vi "Build.vi"(8 "error in (no error)":errorcluster, 11 "Build in":refnum<class "AB_DLL.lvclass">) -> (0 "error out":errorcluster, 1 "GeneratedFiles":path[](array[path]), 2 "GeneratedDirectories":path[](array[path]), 3 "Build out":refnum<class "AB_DLL.lvclass">, 4 "GeneratedFileGUIDs":string[](array[string]), 5 "OutputDirectory":path, 7 "Dependencies":T1[](array[typedef]))   [LabVIEW 2020, in "AB_DLL.lvclass"]
uses:
  <vilib>/AppBuilder/AB_Classes/DLL/AB_DLL.lvclass
  e:/builds/penguin/labview/branches/2020/dev/dist/vi.lib/AppBuilder/AB_Classes/Build/AB_Build.lvclass
  e:/builds/penguin/labview/branches/2020/dev/dist/vi.lib/AppBuilder/AB_Classes/TargetFile/AB_Targetfile.lvclass
  e:/builds/penguin/labview/branches/2020/dev/dist/vi.lib/AppBuilder/AB_Classes/Application/AB_Application.lvclass
  <vilib>/AppBuilder/AB_Dependency.ctl
  <vilib>/Utility/lvfile.llb/LVFileType.ctl
  <vilib>/AppBuilder/AB_Classes/DLL/AB_DLL.lvclass/AB_DLL.ctl
  <vilib>/AppBuilder/Engine/AB_Engine_RTDEP_LibDeploymentInfo.ctl
  <vilib>/AppBuilder/Engine/AB_Engine_RTDEP_Dep_Lib_Info.ctl
  <vilib>/AppBuilder/RW_Project/AB_RW_Project_EXE_ActiveX_Data.ctl
  <resource>/Framework/Providers/Common/provcom_StringGlobals.vi
  <vilib>/AppBuilder/AB_Classes/Application/AB_Application.lvclass
  <vilib>/AppBuilder/AB_Classes/Destination/AB_Destination.lvclass
  <vilib>/AppBuilder/AB_Classes/Build/AB_Build.lvclass
  <vilib>/AppBuilder/AB_Classes/TargetFile/AB_Targetfile.lvclass
  <vilib>/Utility/lvfile.llb/NI_FileType.lvlib
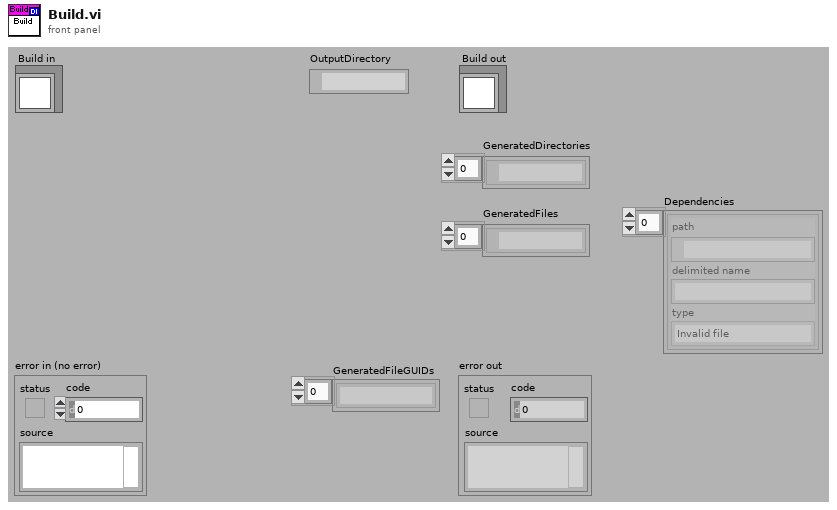
[diagram p1: front panel]
types:
  T1 = typedef "AB_Dependency.ctl" = cluster{"path":path, "delimited name":string, "type":T2}
  T2 = typedef "NI_FileType.lvlib/LVFileType.ctl" = enum32{"Invalid file", "Unknown type", "Instrument", "Control", "Polymorphic VI", "Project", "Library", "LVClass", "XControl", "XNode", "Shared library", ".NET assembly", "ActiveX interface", "CIN", "Run-time menu", "Palette menu", "Help file", "LLB", "XNode Edit Dependency", "Class Private Data Control", "Statechart", "MathScript .m file", "Ladder Diagram", "LVLibp", "XNode Build Dependency"}
  T3 = typedef "AB_Engine_RTDEP_LibDeploymentInfo.ctl" = cluster{"auto undeploy?":bool, "Array":T4[], "hide deployment dialog":bool}
  T4 = typedef "AB_Engine_RTDEP_Dep_Lib_Info.ctl" = cluster{"Library Path":path, "Target Name":string}
  T5 = typedef "AB_RW_Project_EXE_ActiveX_Data.ctl" = cluster{"Major Version":u16, "Minor Version":u16, "ProgID Prefix":string, "Obj CLSIDs":string[], "Enum CLSIDs":string[]}
  T6 = typedef "AB_Build.ctl" = cluster{"buildSpecName":string, "buildSpecDescription":string, "destinations":refnum<class "AB_Destination.lvclass">[], "exclusionOption":T7, "defaultLanguage":string, "supportedLanguages":string[], "excludedDirectories":path[], "buildContext":refnum<vi>, "buildObject":T8, "preview":bool, "programatic":bool, "progressBarEvents":T9, "userLog_Path":path, "preActionID":string, "preAction_Path":path, "postActionID":string, "postAction_Path":path, "eng_checkForBrokenVIs?":bool, "eng_verboseLinkerErrors?":bool, "localDest_Path":path, "targetDest_Path":path, "removeVIObject":u16, "cache":refnum<class "PreviewCache.lvclass">, "use cache":bool, "previewCache_ID":string, "buildCache_ID":string, "eng_TempLocalDest_Path":path, "eng_collectDependencies?":bool, "versionInfo":cluster{"buildVersion":cluster{"major":u16, "minor":u16, "patch":u16, "build":u16}, "autoIncrement":bool}, "eng_enableVIChecksums":bool}
  T7 = typedef "AB_Exclusion_Option.ctl" = cluster{"typedefs":bool, "polymorphicVIs":bool, "unusedLibraryItems":bool, "modifyLibraryFile":bool, "edit-timeDependencies":bool, "inlineVIs":bool, "dependent PPLs":bool, "dependent DLLs":bool}
  T8 = typedef "ItemRef.ctl" = u64
  T9 = typedef "provcom_ProgressBar_Events.ctl" = cluster{"newJob":refnum<user-event>, "newItem":refnum<user-event>, "errorMsg":T10, "cancel":refnum<user-event>}
  T10 = typedef "mxLvBuildError.ctl" = refnum<user-event>
  T11 = typedef "AB_DLL.ctl" = cluster{"delayOSMsg":bool, "includeHeaders":bool, "embeddedRTE":bool, "headerGUID":string, "libGUID":string, "compatibilityWith2011":bool, "includeTypeLibrary":bool, "privateExecutionSystem":bool}
  T12 = typedef "AB_Targetfile.ctl" = cluster{"targetfileName":string, "targetfileGUID":string, "enableDebugging":bool, "versionInfo":cluster{"productName":string, "legalCopyright":string, "companyName":string, "internalName":string, "fileDescription":string}, "eng_consolidatedTypeInfo":string, "fastFileFormat":bool, "eng_LEIFBuildData":u32, "versionIndependent":bool}
  T13 = typedef "AB_Application.ctl" = cluster{"INI_path":path, "INI_itemID":string, "INI_GUID":string, "aliasPath":path, "aliasItemID":string, "aliasGUID":string, "waitDebugging":bool, "copyErrors":bool, "useFFRTE":bool, "includeHWConfig":bool, "showHWConfig":bool, "winsec.certificate":string, "winsec.timestamp":string, "winsec.description":string, "winsec.manifestItemID":string, "winsec.manifestPath":path, "web service itemIDs":string[], "Embedded Server Configuration":T14, "Server Type":enum32{"NI Web Server", "Application Web Server"}}
  T14 = typedef "AB_Embedded_Server_Configuration.ctl" = cluster{"HTTP enabled?":bool, "HTTP port":i32, "HTTPS enabled?":bool, "HTTPS port":i32, "SSL certificate file":path}
  T15 = typedef "AB_Destination.ctl" = cluster{"destName":string, "path":path, "libraryName":string, "preserveHierarchy":bool, "eng_inBuild":bool, "eng_libraryReference":refnum<vi>, "eng_restictAddToNewLibrary":bool}
  T16 = enum32{"invalid OS target", "Mac OS", "Windows 3.1", "Windows 95/NT", "Solaris 1", "Solaris 2", "HP-UX", "PowerMAX", "Linux", "Irix", "Rhapsody", "BeOS", "AIX", "OSF1", "VxWorks", "PharLap", "Carbon", "RTX", "Windows x64", "Linux x64", "Mac OS X x64"}
  T17 = typedef "ABAPI Dist VI Proto Info New.ctl" = cluster{"cptm":string, "params":cluster{"name":string, "dir":enum32{"in", "out", "in/out", "length", "error-out"}, "inputIdx":i32, "outputIdx":i32, "passBy":i32, "lenInput":i32, "lenOutput":i32}[], "callingConv":i32, "name":string, "Description":string, "isCustomDesc":i32}
  T18 = enum32{"invalid CPU target", "Motorola 68K", "PowerPC", "Intel x86", "SPARC", "PA-RISC", "MIPS", "Alpha", "ARM", "AMD/Intel x64"}
  T19 = typedef "AB_Version_Info.ctl" = cluster{"PrivateBuild":string, "SpecialBuild":string, "LegalCopyright":string, "LegalTrademarks":string, "Comments":string, "FileDescription":string, "InternalName":string, "file version":cluster{"major":u16, "minor":u16, "patch":u16, "build":u16}, "ProductName":string, "FileType":u16, "CompanyName":string, "OriginalFilename":string}
  T20 = cluster{"appended path":path, "appended path":path, string, "App Memory Size":u32, "LVRT Target Dialog":i32, "pathAppShell":path, "AppFlags":u32, "activeX info out":T5, "Gen New AX Guids":bool, "defaultLanguage":string, "supportedLanguages":string[], "Lib Deployment Info":T3, "eng_consolidatedTypeInfo":string, "eng_LEIFBuildData":u32}
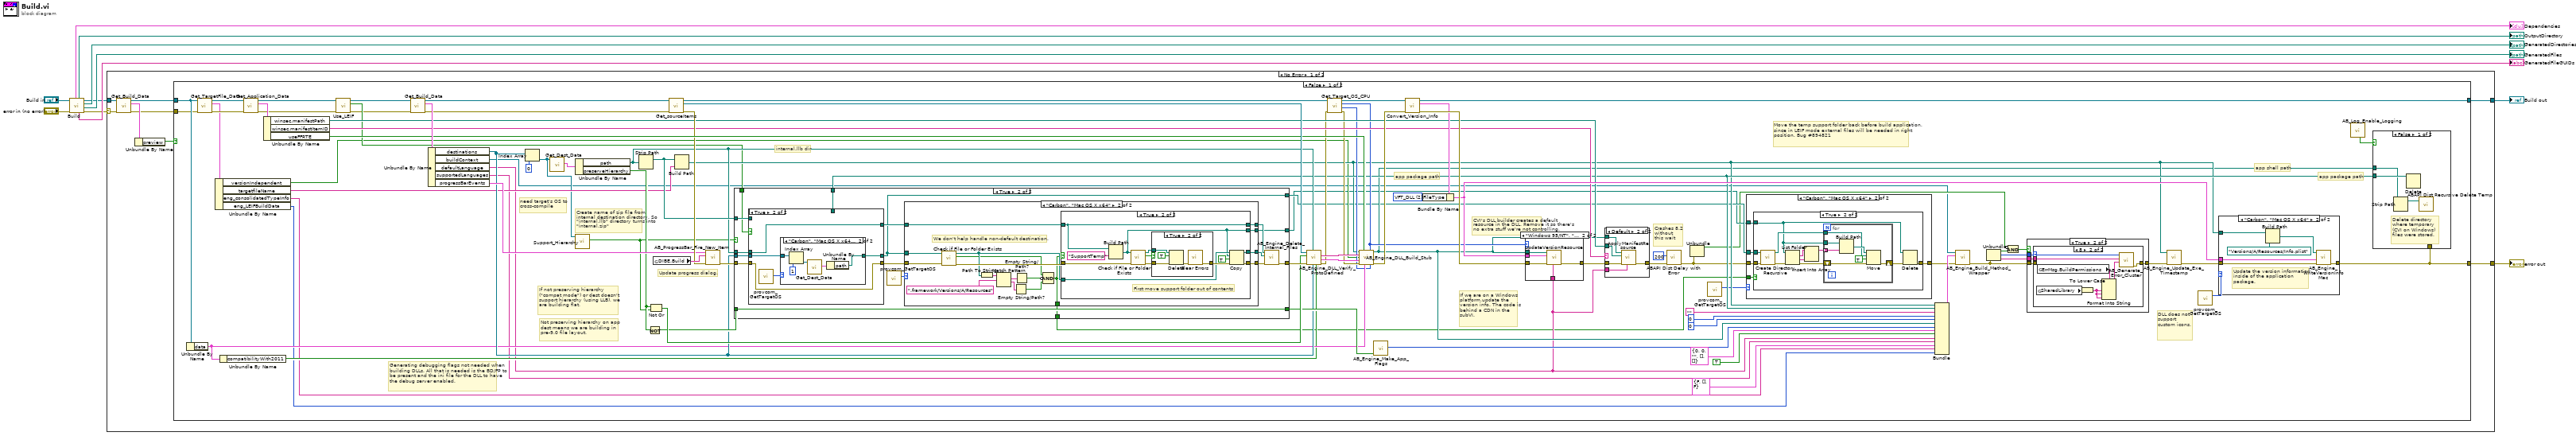
[diagram p0: block diagram]
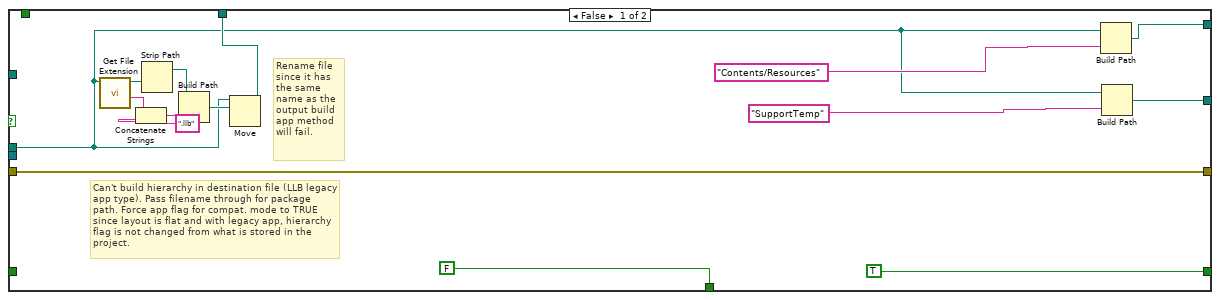
[diagram p6: hidden frame]
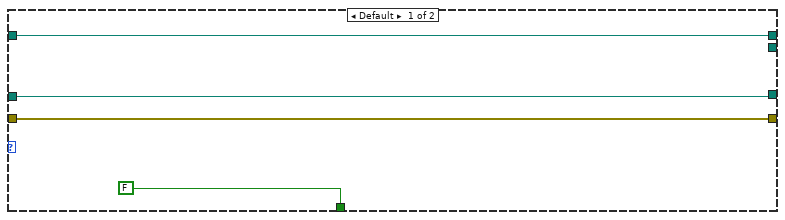
[diagram p7: hidden frame]
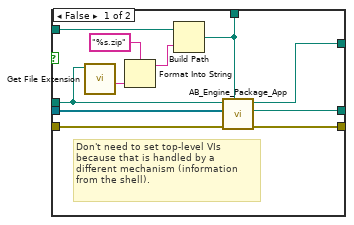
[diagram p10: hidden frame]
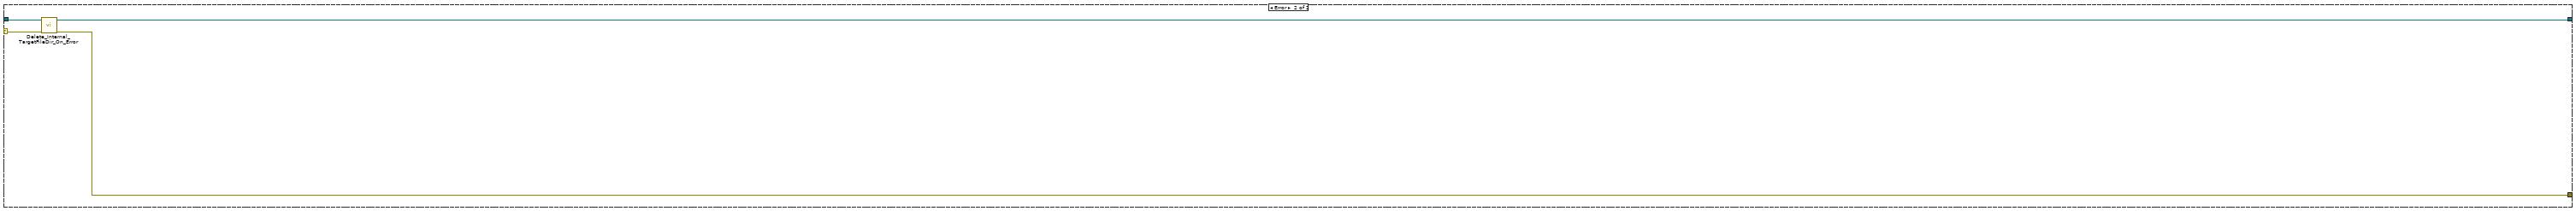
[diagram p17: hidden frame]
diagram:
  n1 = call-parent "Build.vi"("error in (no error)"="error in (no error)", "Build in"="Build in") -> ("error out"=w5:errorcluster, "GeneratedFiles"=→"GeneratedFiles":path[], "GeneratedDirectories"=→"GeneratedDirectories":path[], "Build out"=w4:refnum<class "AB_DLL.lvclass">, "GeneratedFileGUIDs"=→"GeneratedFileGUIDs":string[], "OutputDirectory"=→"OutputDirectory":path, "Dependencies"=→"Dependencies":T1[])  [unwired: 3 out]
  n2 = case shown="No Error" w5 {
    selector: w5 -> [w17 w266]
    tunnel: w4 -> [w18 w268]
    tunnel: [w12 w265] -> w3
    tunnel: [w13 w267] -> w2
    frame No Error {
      n3 = call <vilib>:"Get_Build_Data.vi"("error in (no error)"=w17, "Class in"=w18) -> ("error out"=w15:errorcluster, "data"=w19:T6, "Class out"=w14:refnum<class "AB_DLL.lvclass">)  [unwired: 7 out]
      n4 = Unbundle By Name(w19) -> ("preview"=w16:bool)
      n5 = case shown="False" w16 {
        tunnel: w15 -> [w67 w263]
        tunnel: w14 -> [w69 w264]
        tunnel: [w61 w264] -> w13
        tunnel: [w60 w263] -> w12
        frame False {
          w91 = u16 2 items=["VFT_UNKNOWN", "VFT_APP", "VFT_DLL", "VFT_DRV", "VFT_FONT", "VFT_VXD", "-", "VFT_STATIC_LIB"] ("FileType")
          # "Move the temp support folder back before build application, since in LEIF mode external files will be needed in right position. Bug #894821"
          # "need target's OS to cross-compile"
          # "app shell path"
          # "If not preserving hierarchy (\"compat mode\") or dest doesn't support hierarchy (using LLB), we are building flat."
          # "Not preserving hierarchy on app dest means we are building in pre-9.0 file layout."
          # "Create name of zip file from internal destination directory. So \"internal.llb\" directory turns into \"internal.zip\""
          # "internal.llb dir"
          # "app package path"
          # "app package path"
          # "Update progress dialog."
          # "CVI's DLL builder creates a default resource in the DLL. Remove it so there's no extra stuff we're not controlling."
          # "If we are on a Windows platform,update the version info. The code is behind a CDN in the subVI."
          # "Generating debugging flags not needed when building DLLs. All that is needed is the BD/FP to be present and the ini file for the DLL to have the debug server enabled."
          # "Crashes 8.2 without\nthis wait"
          # "DLL does not support custom icons."
          n6 = Unbundle By Name(w69) -> ("data"=w63:T11)
          n7 = call <vilib>:"Get_TargetFile_Data.vi"("error in (no error)"=w67, "AB_Targetfile in"=w69) -> ("error out"=w66:errorcluster, "data"=w65:T12, "AB_Targetfile out"=w68:refnum<class "AB_DLL.lvclass">)  [unwired: 7 in]
          n8 = Unbundle By Name(w65) -> ("versionIndependent"=w31:bool, "targetfileName"=w64:string, "eng_consolidatedTypeInfo"=w42:string, "eng_LEIFBuildData"=w32:u32)
          n9 = Unbundle By Name(w63) -> ("compatibilityWith2011"=w62:bool)
          n10 = call <vilib>:"Get_Application_Data.vi"("error in (no error)"=w66, "AB_Application in"=w68) -> ("error out"=w34:errorcluster, "data"=w107:T13, "AB_Application out"=w36:refnum<class "AB_DLL.lvclass">)  [unwired: 7 out]
          n11 = Unbundle By Name(w107) -> ("winsec.manifestPath"=w80:path, "winsec.manifestItemID"=w77:string, "useFFRTE"=w97:bool)
          n12 = call <vilib>:"Use_LEIF.vi"("error in (no error)"=w34, "AB_Targetfile in"=w36) -> ("error out"=w33:errorcluster, "use LEIF?"=w37:bool, "AB_Targetfile out"=w35:refnum<class "AB_DLL.lvclass">)  [unwired: 7 in]
          n13 = call <vilib>:"Get_Build_Data.vi"("error in (no error)"=w33, "Class in"=w35) -> ("error out"=w29:errorcluster, "data"=w106:T6, "Class out"=w30:refnum<class "AB_DLL.lvclass">)  [unwired: 7 out]
          n14 = Unbundle By Name(w106) -> ("destinations"=w70:refnum<class "AB_Destination.lvclass">[], "buildContext"=w20:refnum<vi>, "defaultLanguage"=w44:string, "supportedLanguages"=w43:string[], "progressBarEvents"=w88:T9)
          n15 = Index Array(array=w70, index=0) -> (element=w59:refnum<class "AB_Destination.lvclass">)
          n16 = call <vilib>:"Get_Dest_Data.vi"("Class in"=w59) -> ("destName"=w104:T15)  [unwired: 1 in, 9 out]
          n17 = call-dynamic "Support_Hierarchy.vi"("AB_Destination in"=w59) -> ("support hierarchy"=w73:bool)  [unwired: 1 in, 9 out]
          n18 = Unbundle By Name(w104) -> ("path"=w75:path, "preserveHierarchy"=w74:bool)
          n19 = Strip Path(path=w75) -> (stripped path=w81:path)  [unwired: 1 out]
          n20 = Not(x=w74) -> (.not. x?=w72:bool)
          n21 = Not Or(1:w73, 2:w74) -> (0:w76:bool)
          n22 = global read "provcom_StringGlobals.vi" "DIBE.Build"() -> (w90:string)
          n23 = call <vilib>:"Get_sourceItems.vi"("error in (no error)"=w29, "Class in"=w30) -> ("error out"=w89:errorcluster, "sourceItems"=w100:refnum<class "AB_Source.lvclass">[], "Class out"=w58:refnum<class "AB_DLL.lvclass">)  [unwired: 7 out]
          n24 = Build Path(base path=w81, name or relative path=w64) -> (appended path=w50:path)
          n25 = call <vilib>:"AB_ProgressBar_Fire_New_Item.vi"("error in (no error)"=w89, "Label"=w90, "progressBarEvents in"=w88) -> ("error out"=w83:errorcluster)  [unwired: 8 out]
          n26 = case shown="True" w73 {
            tunnel: w83 -> [w159 w176]
            tunnel: [w159 w170] -> w82
            tunnel: w75 -> [w145 w173]
            tunnel: w81 -> [_ w175]
            tunnel: [w151 w174] -> w51
            tunnel: w72 -> [_ w172]
            tunnel: [TRUE w172] -> w71
            tunnel: w70 -> [_ w171]
            tunnel: w37 -> [_ w169]
            tunnel: [w146 w164] -> w25
            tunnel: [w147 w161] -> w26
            tunnel: [FALSE ("file or folder exists?") w160] -> w24
            frame False {
              # "Rename file since it has the same name as the output build app method will fail."
              # "Can't build hierarchy in destination file (LLB legacy app type). Pass filename through for package path. Force app flag for compat. mode to TRUE since layout is flat and with legacy app, hierarchy flag is not changed from what is stored in the project."
              n27 = call <vilib>:"Get File Extension.vi"("file"=w145) -> ("filename without extension"=w157:string, "dup file"=w155:path)  [unwired: 1 in, 8 out]
              n28 = Concatenate Strings(w157, ".llb" ("string")) -> (w154:string)
              n29 = Strip Path(path=w155) -> (stripped path=w153:path)  [unwired: 1 out]
              n30 = Build Path(base path=w153, name or relative path=w154) -> (appended path=w152:path)
              n31 = Move(source path=w145, 10:w152) -> (3:w151:path)  [unwired: 1 in, 4 out]
              n32 = Build Path(base path=w145, name or relative path="Contents/Resources") -> (appended path=w147:path)
              n33 = Build Path(base path=w145, name or relative path="SupportTemp") -> (appended path=w146:path)
            }
            frame True {
              n34 = case shown="True" w169 {
                tunnel: w176 -> [w229 w234]
                tunnel: w175 -> [w225 _]
                tunnel: [w224 _] -> w174
                tunnel: [w221 w234] -> w162
                tunnel: w173 -> [w223 w230]
                tunnel: w171 -> [w222 w232]
                tunnel: [w220 w230] -> w167
                tunnel: [w219 w231] -> w161
                frame False {
                  # "Don't need to set top-level VIs because that is handled by a different mechanism (information from the shell)."
                  n35 = call <vilib>:"Get File Extension.vi"("file"=w223) -> ("filename without extension"=w228:string)  [unwired: 1 in, 9 out]
                  n36 = Format Into String(format string="%s.zip", w228) -> (resulting string=w227:string)  [unwired: 2 in, 1 out]
                  n37 = Build Path(base path=w225, name or relative path=w227) -> (appended path=w224:path)
                  n38 = call <vilib>:"AB_Engine_Package_App.vi"("application package path"=w224, "error in (no error)"=w229, "destinations"=w222, "internal directory"=w223) -> ("error out"=w221:errorcluster, "support dir"=w219:path, "dup internal directory"=w220:path)  [unwired: 1 in, 4 out]
                }
                frame True {
                  n39 = call <resource>:"provcom_GetTargetOS.vi"() -> ("App.TargetOS"=w233:T16)  [unwired: 11 out]
                  n40 = case shown="\"Carbon\", \"Mac OS X x64\"" w233 {
                    tunnel: w232 -> [_ w236]
                    tunnel: [_ w235] -> w231
                    frame Default {
                    }
                    frame "Carbon", "Mac OS X x64" {
                      n41 = Index Array(array=w236, index=1) -> (element=w239:refnum<class "AB_Destination.lvclass">)
                      n42 = call <vilib>:"Get_Dest_Data.vi"("Class in"=w239) -> ("destName"=w238:T15)  [unwired: 1 in, 9 out]
                      n43 = Unbundle By Name(w238) -> ("path"=w235:path)
                    }
                  }
                }
              }
              n44 = call <resource>:"provcom_GetTargetOS.vi"() -> ("App.TargetOS"=w163:T16)  [unwired: 11 out]
              n45 = case shown="\"Carbon\", \"Mac OS X x64\"" w163 {
                tunnel: [w178 w197] -> w168
                tunnel: w167 -> [w180 w196]
                tunnel: [w180 w195] -> w166
                tunnel: [w179 w194] -> w165
                tunnel: [_ w193] -> w164
                tunnel: w162 -> [w178 w192]
                tunnel: w161 -> [w179 w191]
                tunnel: [FALSE ("file or folder exists?") w184] -> w160
                frame Default {
                }
                frame "Carbon", "Mac OS X x64" {
                  # "We don't help handle non-default destination."
                  n46 = call <vilib>:"Check if File or Folder Exists.vi"("error in (no error)"=w192, "path"=w191) -> ("error out"=w190:errorcluster, "file or folder exists?"=w185:bool, "dup path"=w186:path)  [unwired: 7 in]
                  n47 = Path To String(path=w186) -> (string=w189:string)
                  n48 = Match Pattern(string=w189, regular expression=".framework/Versions/A/Resources") -> (match substring=w187:string, after substring=w183:string)  [unwired: 1 in, 2 out]
                  n49 = Empty String/Path?(string/path=w183) -> (empty?=w182:bool)
                  n50 = Empty String/Path?(string/path=w187) -> (empty?=w181:bool)
                  n51 = Compound Arithmetic op=AND(w185, invert w181, w182) -> (w184:bool)
                  n52 = case shown="True" w184 {
                    tunnel: w190 -> [w198 w201]
                    tunnel: w196 -> [w200 w203]
                    tunnel: w186 -> [w199 w206]
                    tunnel: [w199 w205] -> w194
                    tunnel: [w198 w204] -> w197
                    tunnel: [w200 w203] -> w195
                    tunnel: [_ w202] -> w193
                    frame False {
                    }
                    frame True {
                      # "First move support folder out of contents"
                      n53 = Build Path(base path=w203, name or relative path="SupportTemp") -> (appended path=w202:path)
                      n54 = call <vilib>:"Check if File or Folder Exists.vi"("error in (no error)"=w201, "path"=w202) -> ("error out"=w210:errorcluster, "file or folder exists?"=w211:bool, "dup path"=w209:path)  [unwired: 7 in]
                      n55 = case shown="True" w211 {
                        tunnel: w210 -> [w213 w218]
                        tunnel: [w213 w215] -> w208
                        tunnel: w209 -> [_ w214]
                        frame False {
                        }
                        frame True {
                          n56 = Delete(path (use dialog)=w214, entire hierarchy (F)=TRUE, error in=w218) -> (error out=w216:errorcluster)  [unwired: 2 in, 2 out]
                          n57 = call <vilib>:"Clear Errors.vi"("error in (no error)"=w216) -> ("error out"=w215:errorcluster)  [unwired: 5 in, 1 out]
                        }
                      }
                      n58 = Copy(8:w208, 9:TRUE ("overwrite (F)"), 10:w202, 11:w206) -> (0:w204:errorcluster, 3:w205:path)  [unwired: 1 in, 1 out]
                    }
                  }
                }
              }
              n59 = call <vilib>:"AB_Engine_Delete_Internal_Files.vi"("error in (no error)"=w168, "support dir"=w165, "internal directory"=w166) -> ("error out"=w170:errorcluster)  [unwired: 2 in, 6 out]
            }
          }
          n60 = call <vilib>:"AB_Engine_DLL_Verify_ProtoDefined.vi"("compatabilityWIth2011"=w62, "destinations"=w70, "path"=w75, "error in (no error)"=w82, "flat file layout"=w76, "sourceItems"=w100) -> ("error out"=w56:errorcluster, "vipInfo"=w98:T17[], "viNames"=w99:string[])  [unwired: 3 out]
          n61 = call <vilib>:"Get_Target_OS_CPU.vi"("error in (no error)"=w56, "AB_Build in"=w58) -> ("error out"=w55:errorcluster, "Target CPU"=w53:T18, "Target Operating System"=w54:T16, "AB_Build out"=w57:refnum<class "AB_DLL.lvclass">)  [unwired: 6 in]
          n62 = call <vilib>:"AB_Engine_DLL_Build_Stub.vi"("application path"=w50, "useFFRTE"=w97, "Target OS (Windows 95/NT)"=w54, "viNames"=w99, "useBCRTE"=w31, "vipInfo"=w98, "error in (no error)"=w55, "dll data"=w63, "Target CPU"=w53) -> ("pathAppShell"=w46:path, "error out"=w96:errorcluster)  [unwired: 5 in]
          n63 = call <vilib>:"AB_Engine_Make_App_Flags.vi"("App Compatibility Mode"=w71) -> ("AppFlags"=w45:u32)  [unwired: 3 in, 7 out]
          n64 = call-dynamic "Convert_Version_Info.vi"("error in (no error)"=w96, "AB_Targetfile in"=w57) -> ("error out"=w94:errorcluster, "input version info"=w93:T19, "AB_Targetfile out"=w61:refnum<class "AB_DLL.lvclass">)  [unwired: 7 out]
          n65 = Bundle By Name(cluster=w93, "FileType"=w91) -> (w92:T19)
          n66 = case shown="\"Windows 95/NT\", \"Windows x64\"" w54 {
            tunnel: w94 -> [w133 w138]
            tunnel: w92 -> [_ w137]
            tunnel: [w133 w136] -> w79
            tunnel: w44 -> [_ w135]
            tunnel: w46 -> [_ w134]
            frame Default {
            }
            frame "Windows 95/NT", "Windows x64" {
              n67 = call <resource>:"UpdateVersionResource.vi"("default language"=w135, "error in (no error)"=w138, "input version info"=w137, "path"=w134) -> ("error out"=w136:errorcluster)  [unwired: 1 in, 6 out]
            }
          }
          n68 = case shown="Default" w77 {
            tunnel: w80 -> [_ w144]
            tunnel: w46 -> [_ w143]
            tunnel: w79 -> [w139 w142]
            tunnel: [w139 w141] -> w78
            tunnel: w44 -> [_ w140]
            frame "" {
            }
            frame Default {
              n69 = call <resource>:"ApplyManifestResource.vi"("default language"=w140, "error in (no error)"=w142, "manifest path"=w144, "path"=w143) -> ("error out"=w141:errorcluster)  [unwired: 1 in, 6 out]
            }
          }
          n70 = call <vilib>:"ABAPI Dist Delay with Error.vi"("error in (no error)"=w78, "milliseconds to wait"=u32 200) -> ("error out"=w28:errorcluster)  [unwired: 1 in, 8 out]
          n71 = Unbundle(w28) -> ("status"=w21:bool)  [unwired: 2 out]
          n72 = call <resource>:"provcom_GetTargetOS.vi"() -> ("App.TargetOS"=w22:T16)  [unwired: 11 out]
          n73 = case shown="\"Carbon\", \"Mac OS X x64\"" w22 {
            tunnel: w28 -> [w108 w113]
            tunnel: [w108 w112] -> w27
            tunnel: w25 -> [_ w111]
            tunnel: w26 -> [_ w110]
            tunnel: w24 -> [_ w109]
            frame "invalid OS target", Default {
            }
            frame "Carbon", "Mac OS X x64" {
              n74 = case shown="True" w109 {
                tunnel: w113 -> [w114 w125]
                tunnel: [w114 w120] -> w112
                tunnel: w111 -> [_ w115]
                tunnel: w110 -> [_ w117]
                frame False {
                }
                frame True {
                  n75 = call <vilib>:"Create Directory Recursive.vi"("error in (no error)"=w125, "directory"=w117) -> ("error out"=w118:errorcluster, "directory copy"=w116:path)  [unwired: 3 in, 1 out]
                  n76 = List Folder(path=w115, error in=w118) -> (filenames=w123:string[], folder names=w124:string[], error out=w122:errorcluster)  [unwired: 2 in, 1 out]
                  n77 = Insert Into Array(array=w123, new element=w124) -> (w119:string[])  [unwired: 1 in]
                  n78 = for {
                    shift-right: [w129] -> w121
                    shift-left: w122 -> [w132]
                    tunnel: w119 -> [w131] mode=indexing
                    tunnel: w115 -> [w130]
                    tunnel: w116 -> [w126]
                    n79 = Build Path(base path=w130, name or relative path=w131) -> (appended path=w127:path)
                    n80 = Move(source path=w127, error in=w132, 9:TRUE ("overwrite (F)"), 10:w126) -> (error out=w129:errorcluster)  [unwired: 1 in, 2 out]
                  }
                  n81 = Delete(path (use dialog)=w115, error in=w121) -> (error out=w120:errorcluster)  [unwired: 3 in, 2 out]
                }
              }
            }
          }
          n82 = Bundle("appended path"=w50, "appended path"=w51, "", "App Memory Size"=u32 0, "LVRT Target Dialog"=0, "pathAppShell"=w46, "AppFlags"=w45, "activeX info out"=T5 {"Major Version"=0, "Minor Version"=0, "ProgID Prefix"="", "Obj CLSIDs"=[], "Enum CLSIDs"=[]}, "Gen New AX Guids"=TRUE, "defaultLanguage"=w44, "supportedLanguages"=w43, "Lib Deployment Info"=T3 {"auto undeploy?"=FALSE, "Array"=[], "hide deployment dialog"=FALSE}, "eng_consolidatedTypeInfo"=w42, "eng_LEIFBuildData"=w32) -> (w41:T20)  [unwired: 1 in]
          n83 = call <vilib>:"AB_Engine_Build_Method_Wrapper.vi"("error in"=w27, "build cluster"=w41, "buildContext"=w20) -> ("error out"=w52:errorcluster)  [unwired: 7 in, 1 out]
          n84 = Unbundle(w52) -> ("status"=w84:bool, "code"=w86:i32, "source"=w87:string)
          n85 = Compound Arithmetic op=AND(invert w21, w84) -> (w85:bool)
          n86 = case shown="True" w85 {
            tunnel: w52 -> [w240 w243]
            tunnel: w86 -> [_ w244]
            tunnel: [w240 w242] -> w23
            tunnel: w87 -> [_ w241]
            frame False {
            }
            frame True {
              n87 = case shown="8" w244 {
                selector: w244 -> [_ w252]
                tunnel: w243 -> [w245 _]
                tunnel: [w245 w250] -> w242
                tunnel: w241 -> [_ w251]
                frame Default {
                }
                frame 8 {
                  n88 = global read "provcom_StringGlobals.vi" "SharedLibrary"() -> (w247:string)
                  n89 = global read "provcom_StringGlobals.vi" "ErrMsg.BuildPermissions"() -> (w248:string)
                  n90 = To Lower Case(string=w247) -> (all lower case string=w249:string)
                  n91 = Format Into String(format string=w248, w249, w249, w249) -> (resulting string=w246:string)  [unwired: 2 in, 1 out]
                  n92 = call <vilib>:"AB_Generate_Error_Cluster.vi"("Additional Message"=w246, "source"=w251, "Code"=w252) -> ("error out"=w250:errorcluster)  [unwired: 1 in, 7 out]
                }
              }
            }
          }
          n93 = call <vilib>:"AB_Engine_Update_Exe_Timestamp.vi"("error in (no error)"=w23, "pathExe"=w50) -> ("error out"=w102:errorcluster)  [unwired: 9 out]
          n94 = call <resource>:"provcom_GetTargetOS.vi"() -> ("App.TargetOS"=w95:T16)  [unwired: 11 out]
          n95 = case shown="\"Carbon\", \"Mac OS X x64\"" w95 {
            tunnel: w102 -> [w253 w258]
            tunnel: [w253 w254] -> w60
            tunnel: w92 -> [_ w257]
            tunnel: w50 -> [_ w255]
            frame "invalid OS target", Default {
            }
            frame "Carbon", "Mac OS X x64" {
              # "Update the version information inside of the application package."
              n96 = Build Path(base path=w255, name or relative path=path "Versions/A/Resources/Info.plist") -> (appended path=w259:path)
              n97 = call <vilib>:"AB_Engine_WriteVersionInfoMac.vi"("error in (no error)"=w258, "version info"=w257, "FilePath"=w259) -> ("error out"=w254:errorcluster)  [unwired: 1 in, 7 out]
            }
          }
          n98 = call <vilib>:"AB_Log_Enable_Logging.vi"() -> ("keep internal.llb"=w103:bool)  [unwired: 2 in, 9 out]
          n99 = case shown="False" w103 {
            tunnel: w60 -> [_ _]
            tunnel: w51 -> [w262 _]
            tunnel: w46 -> [w260 _]
            frame False {
              # "Delete directory where temporary (CVI on Windows) files were stored."
              n100 = Strip Path(path=w260) -> (stripped path=w261:path)  [unwired: 1 out]
              n101 = Delete(path (use dialog)=w262) -> ()  [unwired: 1 in, 6 out]
              n102 = call <vilib>:"ABAPI Dist Recursive Delete Temp.vi"("path"=w261) -> ()  [unwired: 1 in, 2 out]
            }
            frame True {
            }
          }
        }
        frame True {
        }
      }
    }
    frame Error {
      n103 = call-dynamic "Delete_Internal_TargetFileDir_On_Error.vi"("error in (no error)"=w266, "Build in"=w268) -> ("error out"=w265:errorcluster, "Build out"=w267:refnum<class "AB_DLL.lvclass">)  [unwired: 8 in]
    }
  }
  "error out" <- w3
  "Build out" <- w2
